vi "Set Sample Rate.vi"(8 "error in (no error)":errorcluster, 10 "Sample Rate":u32, 11 "RTL-SDR in":refnum<class "RTL-SDR.lvclass">) -> (0 "error out":errorcluster, 1 "function return":i32, 3 "RTL-SDR out":refnum<class "RTL-SDR.lvclass">)   [LabVIEW 2015, in "RTL-SDR.lvclass"]
uses:
  RTL-SDR.lvclass
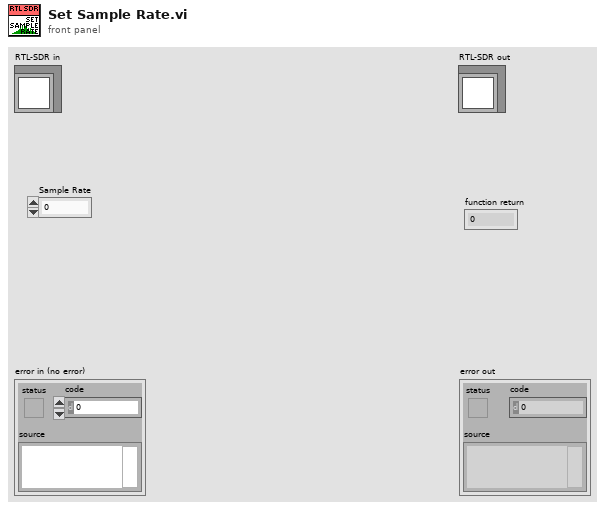
[diagram p1: front panel]
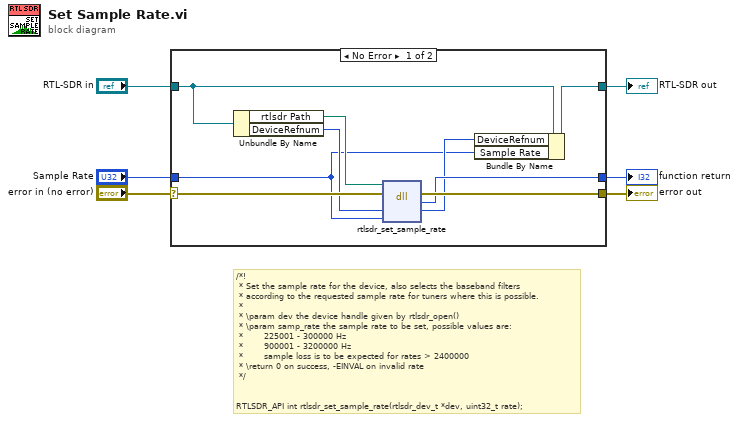
[diagram p0: block diagram]
diagram:
  # "/*!\n * Set the sample rate for the device, also selects the baseband filters\n * according to the requested sample rate for tuners where this is possible.\n *\n * \\param dev the device handle given by rtlsdr_open()\n * \\param samp_rate the sample rate to be set, possible values are:\n * \t\t    225001 - 300000 Hz\n * \t\t    900001 - 3200000 Hz\n * \t\t    sample loss is to be expected for rates > 2400000\n * \\return 0 on success, -EINVAL on invalid rate\n */\n\n\nRTLSDR_API int rtlsdr_set_sample_rate(rtlsdr_dev_t *dev, uint32_t rate);"
  n1 = case shown="No Error" "error in (no error)" {
    selector: "error in (no error)" -> [w15 w17]
    tunnel: [w14 w17] -> w5
    tunnel: [w10 w16] -> w3
    tunnel: "RTL-SDR in" -> [w13 w16]
    tunnel: [w9 _] -> w2
    tunnel: "Sample Rate" -> [w7 _]
    frame No Error {
      n2 = Unbundle By Name(w13) -> ("rtlsdr Path"=w11:path, "DeviceRefnum"=w12:u64)
      n3 = dll-call lib="C:/Users/Ivan/Desktop/D-23-09-24 (RTL-SDR)/Project (Pelleng-SDR)/rtlsdr/dll/rtlsdr.*" fn="rtlsdr_set_sample_rate"(path in=w11, error in=w15, "DeviceRefnum"=w12, "Sample Rate"=w7) -> (error out=w14:errorcluster, "return type"=w9:i32, "DeviceRefnum"=w8:u64)  [unwired: 2 in, 1 out]
      n4 = Bundle By Name(cluster=w13, "DeviceRefnum"=w8, "Sample Rate"=w7) -> (w10:refnum<class "RTL-SDR.lvclass">)
    }
    frame Error {
    }
  }
  "error out" <- w5
  "RTL-SDR out" <- w3
  "function return" <- w2
